vi "Utility Unit Info.vi"(7 "Action":T2(ring), 8 "Error In (no error)":errorcluster, 10 "Unit Info In":T1={"ID String"="", "Model"="", "Model #"=-1, "# Channels"=-1, "Options"="", "Firmware"="", "FPGA Ver"=""}, 11 "VISA resource name in":refnum<visa-resource-name>) -> (0 "Error Out":errorcluster, 1 "Unit Info Out":T1={"ID String"="", "Model"="", "Model #"=-1, "# Channels"=-1, "Options"="", "Firmware"="", "FPGA Ver"=""}, 3 "VISA resource name out":refnum<visa-resource-name>)   [LabVIEW 2020, in "Berkeley Nucleonics 500 Series.lvlib"]
doc: "This VI stores information about the unit connected via a given VISA session. It is private in scope and should only be written to by the Initialize VI."
uses:
  Berkeley Nucleonics 500 Series.lvlib
  Unit Info.ctl
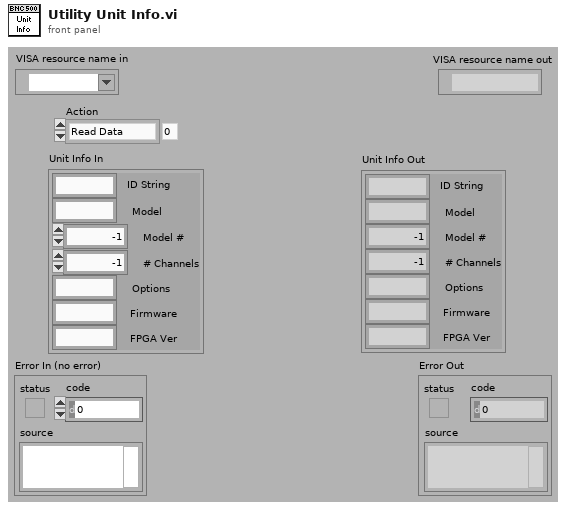
[diagram p1: front panel]
types:
  T1 = typedef "Berkeley Nucleonics 500 Series.lvlib/Unit Info.ctl" = cluster{"ID String":string, "Model":string, "Model #":i32, "# Channels":i32, "Options":string, "Firmware":string, "FPGA Ver":string}
  T2 = enum16{"Read Data", "Write Data", "Dispose of Data", "Clear ALL Data"}
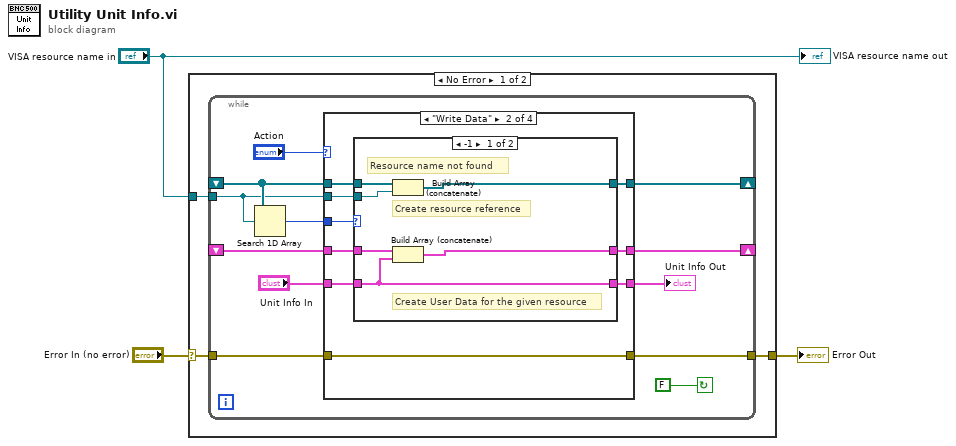
[diagram p0: block diagram]
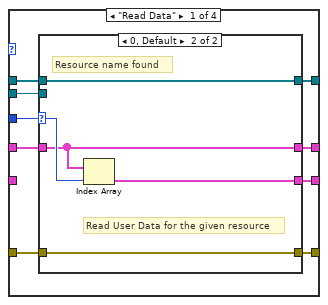
[diagram p2: hidden frame]
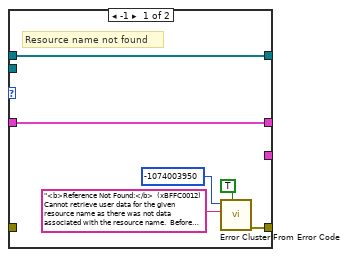
[diagram p3: hidden frame]
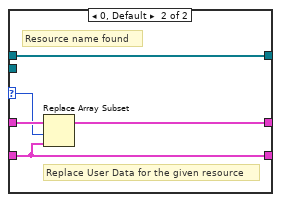
[diagram p4: hidden frame]
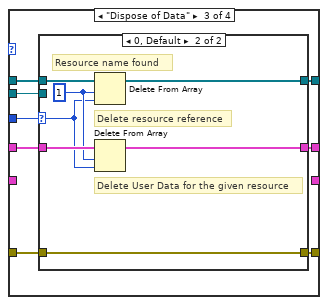
[diagram p5: hidden frame]
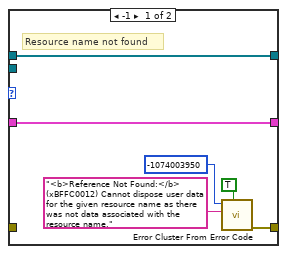
[diagram p6: hidden frame]
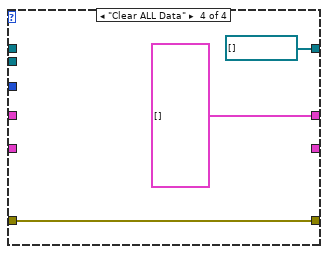
[diagram p7: hidden frame]
diagram:
  n1 = case shown="No Error" "Error In (no error)" {
    selector: "Error In (no error)" -> [w5 w83]
    tunnel: "VISA resource name in" -> [w6 _]
    tunnel: [w4 w83] -> w1
    frame No Error {
      n2 = while {
        shift-right: [w14] -> _
        shift-left: _ -> [w15]
        shift-right: [w17] -> _
        shift-left: _ -> [w18]
        tunnel: w6 -> [w13]
        tunnel: w5 -> [w10]
        tunnel: [w9] -> w4
        stop <- FALSE continue-if-true
        n3 = Search 1D Array(1D array=w15, element=w13) -> (index of element=w16:i32)  [unwired: 1 in]
        n4 = case shown="\"Write Data\"" "Action" {
          tunnel: w18 -> [w27 w47 w66 _]
          tunnel: [w26 w46 w65 T1[] []] -> w17
          tunnel: w16 -> [w25 w45 w64 _]
          tunnel: w15 -> [w24 w44 w63 _]
          tunnel: [w23 w43 w62 refnum<visa-resource-name>[] []] -> w14
          tunnel: w13 -> [w22 w42 w61 _]
          tunnel: w10 -> [w20 w39 w59 w82]
          tunnel: [w21 w39 w60 w82] -> w9
          tunnel: [w19 w41 _ _] -> w8
          tunnel: "Unit Info In" -> [_ w40 _ _]
          frame "Read Data" {
            n5 = case shown="0, Default" w25 {
              selector: w25 -> [_ w38]
              tunnel: [w32 w36] -> w26
              tunnel: w27 -> [w32 w36]
              tunnel: w24 -> [w33 w37]
              tunnel: [w33 w37] -> w23
              tunnel: w22 -> [_ _]
              tunnel: [w31 w35] -> w21
              tunnel: w20 -> [_ w35]
              tunnel: [_ w34] -> w19
              frame -1 {
                # "Resource name not found"
                n6 = call <vilib>:"Error Cluster From Error Code.vi"("show call chain? (False)"=TRUE, "error message (\"\")"="<b>Reference Not Found:</b>  (xBFFC0012) Cannot retrieve user data for the given resource name as there was not data associated with the resource name.  Before you can read data, you need to write the user data using the Write Data action of this User Data VI. ", "error code (0)"=-1074003950 ("Code")) -> ("error out"=w31:errorcluster)  [unwired: 6 in]
              }
              frame 0, Default {
                # "Read User Data for the given resource"
                # "Resource name found"
                n7 = Index Array(array=w36, index=w38) -> (element=w34:T1)
              }
            }
          }
          frame "Write Data" {
            n8 = case shown="-1" w45 {
              selector: w45 -> [_ w56]
              tunnel: [w51 w58] -> w46
              tunnel: w47 -> [w52 w57]
              tunnel: w44 -> [w53 w55]
              tunnel: [w49 w55] -> w43
              tunnel: w42 -> [w50 _]
              tunnel: w40 -> [w48 w54]
              tunnel: [w48 w54] -> w41
              frame -1 {
                # "Create resource reference"
                # "Create User Data for the given resource"
                # "Resource name not found"
                n9 = Build Array (concatenate)(w53, w50) -> (w49:refnum<visa-resource-name>[])
                n10 = Build Array (concatenate)(w52, w48) -> (w51:T1[])
              }
              frame 0, Default {
                # "Replace User Data for the given resource"
                # "Resource name found"
                n11 = Replace Array Subset(array=w57, new element=w54, index=w56) -> (w58:T1[])
              }
            }
          }
          frame "Dispose of Data" {
            n12 = case shown="0, Default" w64 {
              selector: w64 -> [_ w73]
              tunnel: [w71 w79] -> w65
              tunnel: w66 -> [w71 w78]
              tunnel: w63 -> [w72 w76]
              tunnel: [w72 w75] -> w62
              tunnel: w61 -> [_ _]
              tunnel: [w70 w77] -> w60
              tunnel: w59 -> [_ w77]
              frame -1 {
                # "Resource name not found"
                n13 = call <vilib>:"Error Cluster From Error Code.vi"("show call chain? (False)"=TRUE, "error message (\"\")"="<b>Reference Not Found:</b>  (xBFFC0012) Cannot dispose user data for the given resource name as there was not data associated with the resource name.", "error code (0)"=-1074003950 ("Code")) -> ("error out"=w70:errorcluster)  [unwired: 6 in]
              }
              frame 0, Default {
                w74 = 1 ("length")
                # "Delete resource reference"
                # "Delete User Data for the given resource"
                # "Resource name found"
                n14 = Delete From Array(array=w76, length=w74, index=w73) -> (array with subset deleted=w75:refnum<visa-resource-name>[])  [unwired: 1 out]
                n15 = Delete From Array(array=w78, length=w74, index=w73) -> (array with subset deleted=w79:T1[])  [unwired: 1 out]
              }
            }
          }
          frame "Clear ALL Data" {
          }
        }
        "Unit Info Out" <- w8
      }
    }
    frame Error {
    }
  }
  "Error Out" <- w1
  "VISA resource name out" <- "VISA resource name in"
